vi "call check convergence.vi"(0 "f":dbl, 1 "current iteration":i32, 5 "X":dbl[](array[numeric]), 7 "gradient":dbl[](array[numeric]), 9 "number of function evaluations":i32, 11 "error in":errorcluster, 12 "vi reference":refnum<vi>, 14 "stopping criteria":T1={"function tolerance"=1e-06, "parameter tolerance"=1e-06, "max iterations"=0, "max function calls"=0, "gradient tolerance"=0.0, "max time (sec)"=1000.0, "initial tick count"=0}) -> (3 "line search tol":dbl, 4 "stop?":bool, 6 "ftol":dbl, 10 "xtol":dbl, 15 "error out":errorcluster)   [LabVIEW 2014, in "NI_Gmath.lvlib"]
uses:
  NI_Gmath.lvlib
  stopping criteria with time.ctl
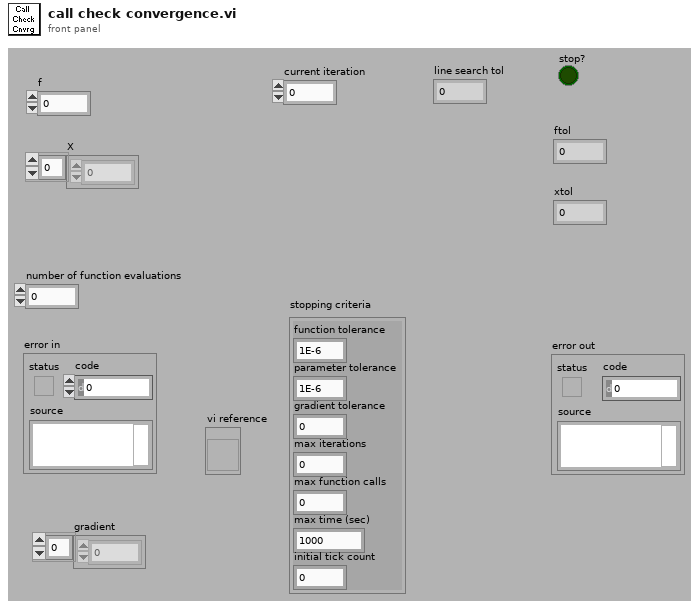
[diagram p1: front panel]
types:
  T1 = typedef "NI_Gmath.lvlib/stopping criteria with time.ctl" = cluster{"function tolerance":dbl, "parameter tolerance":dbl, "max iterations":i32, "max function calls":i32, "gradient tolerance":dbl, "max time (sec)":dbl, "initial tick count":u32}
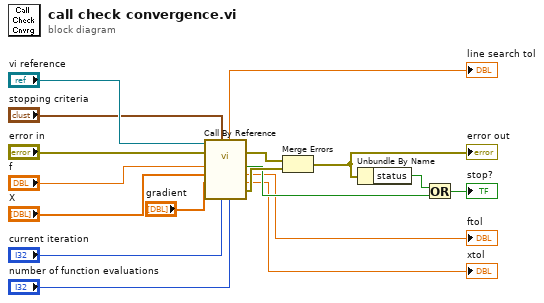
[diagram p0: block diagram]
diagram:
  n1 = call-by-ref "?"(reference="vi reference", error in="error in", "number of function evaluations"="number of function evaluations", "current iteration"="current iteration", "stopping criteria"="stopping criteria", "gradient"="gradient", "X"="X", "f"="f") -> (error out=w13:errorcluster, 0:"error out"=w9:errorcluster, "xtol"=→"xtol":dbl, "ftol"=→"ftol":dbl, "stop?"=w8:bool, "line search tol"=→"line search tol":dbl)  [unwired: 1 in, 1 out]
  n2 = Merge Errors(w13, w9) -> (w12:errorcluster)
  "error out" <- w12
  n3 = Unbundle By Name(w12) -> ("status"=w15:bool)
  n4 = Or(x=w15, y=w8) -> (x .or. y?=→"stop?":bool)
